vi "Simple Reader.vi"(8 "error in (no error)":errorcluster, 11 "Micron Optics Driver in":refnum<class "Micron Optics Driver.lvclass">) -> (0 "error out":errorcluster, 2 "Signals":dbl[](array[numeric]), 3 "Micron Optics Driver out":refnum<class "Micron Optics Driver.lvclass">)   [LabVIEW 2016, in "Micron Optics Driver.lvclass"]
uses:
  Micron Optics Driver.lvclass
  C:/github/NHMFL_Core/Libraries/Instruments/Instrument Driver/Instrument Driver.lvclass
  Instrument Driver/Instrument Driver.lvclass/Instrument Driver.ctl
  Instrument Driver/Read Recorder name.vi
  Instrument Driver/Write Channel names.vi
  Instrument Driver/Write Channel units.vi
  Read Micron Configuration.vi
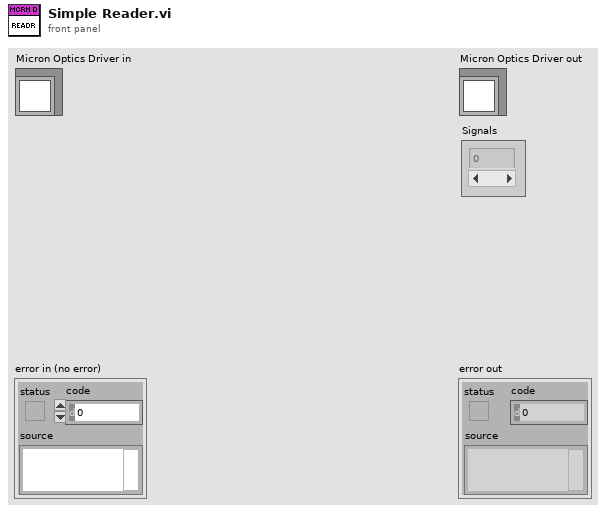
[diagram p1: front panel]
types:
  T1 = typedef "Micron optics configuration.ctl" = cluster{"Reference channel":i32, "Detection Setting IDs":u8[], "Address":string, "Stream and average":bool}
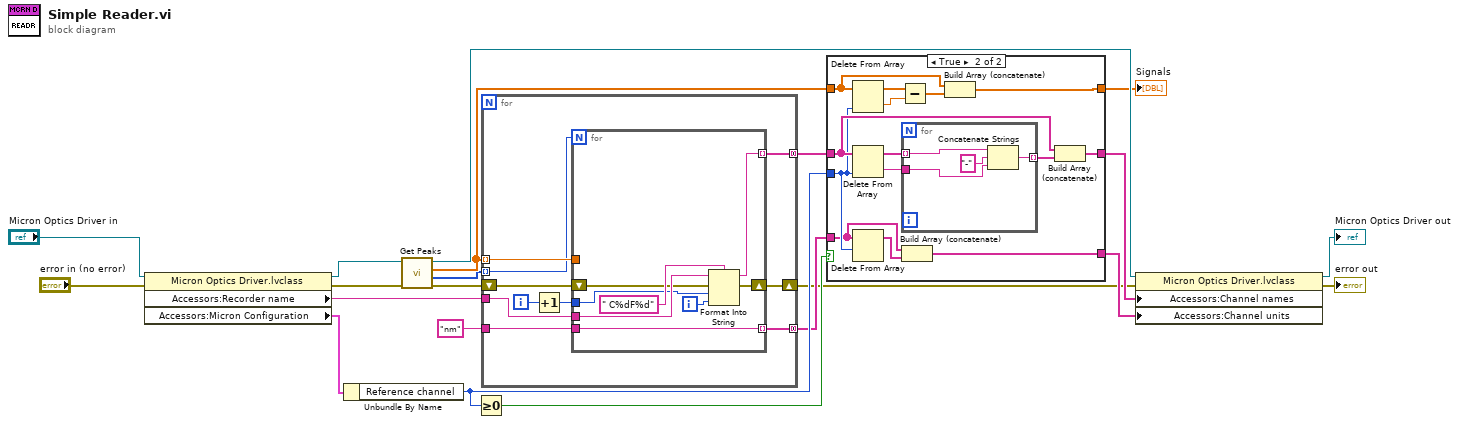
[diagram p0: block diagram]
diagram:
  n1 = property class="Micron Optics Driver.lvclass"(reference="Micron Optics Driver in", error in="error in (no error)") -> (reference out=w21:refnum<class "Micron Optics Driver.lvclass">, error out=w17:errorcluster, "Accessors:Recorder name"=w20:string, "Accessors:Micron Configuration"=w12:T1)
  n2 = Unbundle By Name(w12) -> ("Reference channel"=w9:i32)
  n3 = call-dynamic "Get Peaks.vi"("error in (no error)"=w17, "Micron Optics Driver in"=w21) -> ("error out"=w2:errorcluster, "Peaks per channel"=w3:i32[], "Peaks"=w11:dbl[], "Micron Optics Driver out"=w18:refnum<class "Micron Optics Driver.lvclass">)  [unwired: 6 in]
  n4 = Greater Or Equal To 0?(x=w9) -> (x >= 0?=w10:bool)
  n5 = for {
    tunnel: w20 -> [w31]
    tunnel: "nm" -> [w30]
    tunnel: w11 -> [w29] mode=indexing
    tunnel: [w28] -> w8 mode=concatenating
    tunnel: [w27] -> w5 mode=concatenating
    tunnel: w3 -> [w26] mode=indexing
    shift-right: [w22] -> w1
    shift-left: w2 -> [w23]
    i -> [w25]
    n6 = Increment(x=w25) -> (x+1=w24:i32)
    n7 = for {
      N: w26 -> [_]
      tunnel: w29 -> [_]
      tunnel: [w38] -> w28 mode=indexing
      tunnel: w31 -> [w37]
      tunnel: w30 -> [w36]
      tunnel: [w36] -> w27 mode=indexing
      tunnel: w24 -> [w34]
      shift-right: [w32] -> w22
      shift-left: w23 -> [w33]
      i -> [w35]
      n8 = Format Into String(format string=" C%dF%d", initial string=w37, error in=w33, w34, w35) -> (resulting string=w38:string, error out=w32:errorcluster)
    }
  }
  n9 = case shown="True" w10 {
    tunnel: w11 -> [w41 w49]
    tunnel: w9 -> [_ w46]
    tunnel: w8 -> [w42 w52]
    tunnel: [w42 w50] -> w7
    tunnel: [w41 w47] -> w6
    tunnel: w5 -> [w40 w44]
    tunnel: [w40 w43] -> w4
    frame False {
    }
    frame True {
      n10 = Delete From Array(array=w49, index=w46) -> (deleted portion=w55:dbl, array with subset deleted=w56:dbl[])  [unwired: 1 in]
      n11 = Delete From Array(array=w52, index=w46) -> (deleted portion=w53:string, array with subset deleted=w54:string[])  [unwired: 1 in]
      n12 = Delete From Array(array=w44, length=w46) -> (array with subset deleted=w45:string[])  [unwired: 1 in, 1 out]
      n13 = Subtract(x=w56, y=w55) -> (x-y=w48:dbl[])
      n14 = for {
        tunnel: w54 -> [w60] mode=indexing
        tunnel: w53 -> [w59]
        tunnel: [w57] -> w51 mode=indexing
        n15 = Concatenate Strings(w60, "-" ("string"), w59) -> (w57:string)
      }
      n16 = Build Array (concatenate)(w44, w45) -> (w43:string[])
      n17 = Build Array (concatenate)(w49, w48) -> (w47:dbl[])
      n18 = Build Array (concatenate)(w52, w51) -> (w50:string[])
    }
  }
  "Signals" <- w6
  n19 = property class="Micron Optics Driver.lvclass"(reference=w18, error in=w1, "Accessors:Channel names"=w7, "Accessors:Channel units"=w4) -> (reference out=→"Micron Optics Driver out":refnum<class "Micron Optics Driver.lvclass">, error out=→"error out":errorcluster)
